vi "Phasor Explorer Refresh Settings.vi"(8 "error in (no error)":errorcluster, 11 "VI in":refnum<vi>) -> (0 "error out":errorcluster)   [LabVIEW 2019]
uses:
  Phasor Explorer Phasor Parameters.ctl
  Phasor Calculation Type.ctl
  SEPL Type.ctl
  Phasor Explorer Gate Parameters.ctl
  Gate Type.ctl
  Type of User-defined Function.ctl
  Phasor Explorer Decay Parameters.ctl
  IRF Model.ctl
  Phasor Explorer Display Parameters.ctl
  Type of Series.ctl
panel:
  in  "Display Parameters":T1={"# Points"=1, "Ramp Type"=enum."Linear", "Type of Series"=enum."1-Exp Decays", "Min tau"=0.0, "Max tau"=0.0, "Include 0"=FALSE, "Include Infinity"=FALSE} {"Min tau" min=0.0; "Max tau" min=0.0; "# Points" min=1 step=1}
  in  "Decay & IRF Parameters":T3 {"Lifetime" min=0.0; "IRF Period" min=0.0}
  in  "Gate Parameters":T5={"First Gate Start"=0.0, "Use Gate Center"=FALSE, "Gate Width"=0.0, "Gate Step"=0.0, "# Gates"=1.0, "Gate Type"=enum."Square", "Edge Width"=0.0, "Top Slope"=0.0, "Reversed Sawtooth?"=FALSE, "Analytical Computation"=FALSE, "Integration"=enum."Item 0", "Tolerance"=1.0, "# Steps"=1.0, "Type of User-defined Function"=enum."Gate", "Use Gate Step"=FALSE} {"# Steps" min=0.0; "Tolerance" min=0.0; "Top Slope" min=0.0; "Edge Width" min=0.0; "Gate Step" min=0.0; "# Gates" min=1.0 step=1.0; "Gate Width" min=0.0}
  in  "Phasor Parameters":T8={"Harmonic Frequency"=0.0, "Use f* = 1/D Frequency"=FALSE, "Calibrated Phasor"=FALSE, "Calibration Lifetime"=1e-09, "Phasor Calculation"=enum."Direct Sum", "SEPL Type"=enum."UC", "# Gates"=1.0, "Square Gate Width"=1e-09, "Show Ticks"=FALSE} {"Square Gate Width" min=0.0; "# Gates" min=0.0; "Calibration Lifetime" min=0.0; "Harmonic Frequency" min=0.0}
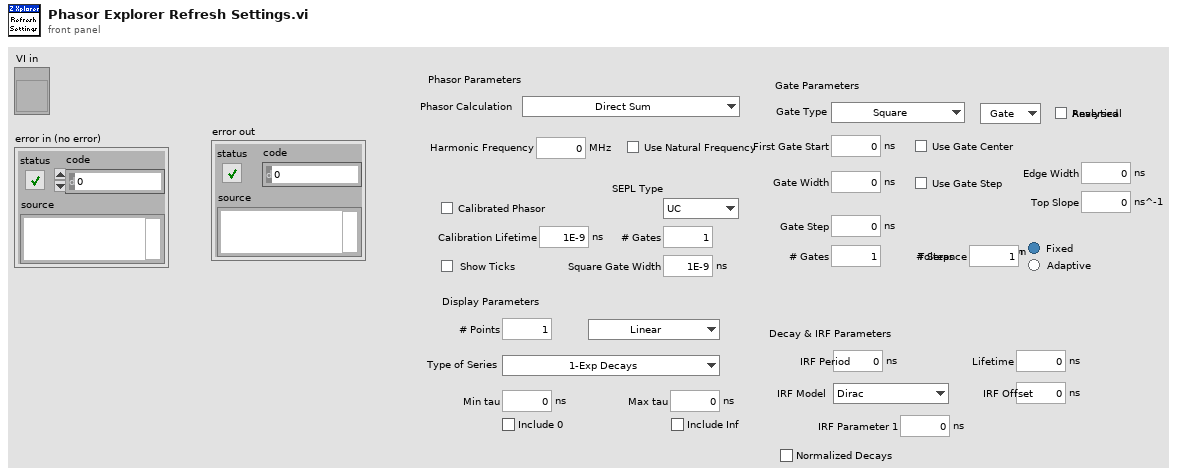
[diagram p1: front panel]
types:
  T1 = typedef "Phasor Explorer Display Parameters.ctl" = cluster{"# Points":i32, "Ramp Type":enum16{"Linear", "Logarithmic"}, "Type of Series":T2, "Min tau":dbl[unit], "Max tau":dbl[unit], "Include 0":bool, "Include Infinity":bool}
  T2 = typedef "Type of Series.ctl" = enum16{"1-Exp Decays", "Linear Combination of 1-Exp"}
  T3 = typedef "Phasor Explorer Decay Parameters.ctl" = cluster{"Lifetime":dbl[unit], "IRF Offset":dbl[unit], "IRF Period":dbl[unit], "Normalized Decays":bool, "IRF Model":T4, "IRF Parameter 1":dbl[unit]}
  T4 = typedef "IRF Model.ctl" = enum16{"Dirac", "Exponential"}
  T5 = typedef "Phasor Explorer Gate Parameters.ctl" = cluster{"First Gate Start":dbl[unit], "Use Gate Center":bool, "Gate Width":dbl[unit], "Gate Step":dbl[unit], "# Gates":dbl, "Gate Type":T6, "Edge Width":dbl[unit], "Top Slope":dbl[unit], "Reversed Sawtooth?":bool, "Analytical Computation":bool, "Integration":enum32{"Item 0", "Item 1"}, "Tolerance":dbl, "# Steps":dbl, "Type of User-defined Function":T7, "Use Gate Step":bool}
  T6 = typedef "Gate Type.ctl" = enum16{"Square", "Finite Edge Square", "Finite Edge, Tilted Top Square", "Triangle", "Sawtooth", "User-defined"}
  T7 = typedef "Type of User-defined Function.ctl" = enum16{"Gate", "IRF"}
  T8 = typedef "Phasor Explorer Phasor Parameters.ctl" = cluster{"Harmonic Frequency":dbl[unit], "Use f* = 1/D Frequency":bool, "Calibrated Phasor":bool, "Calibration Lifetime":dbl[unit], "Phasor Calculation":T9, "SEPL Type":T10, "# Gates":dbl, "Square Gate Width":dbl[unit], "Show Ticks":bool}
  T9 = typedef "Phasor Calculation Type.ctl" = enum16{"Direct Sum", "Analytical Formula"}
  T10 = typedef "SEPL Type.ctl" = enum16{"UC", "L_N", "L_N[W]", "L_X"}
  T11 = typedef "Phasor Explorer Settings List.ctl" = enum16{"Display Parameters", "Phasor Parameters", "Decay & IRF Parameters", "Gate Parameters", "Detector Parameters", "f*", "tau*"}
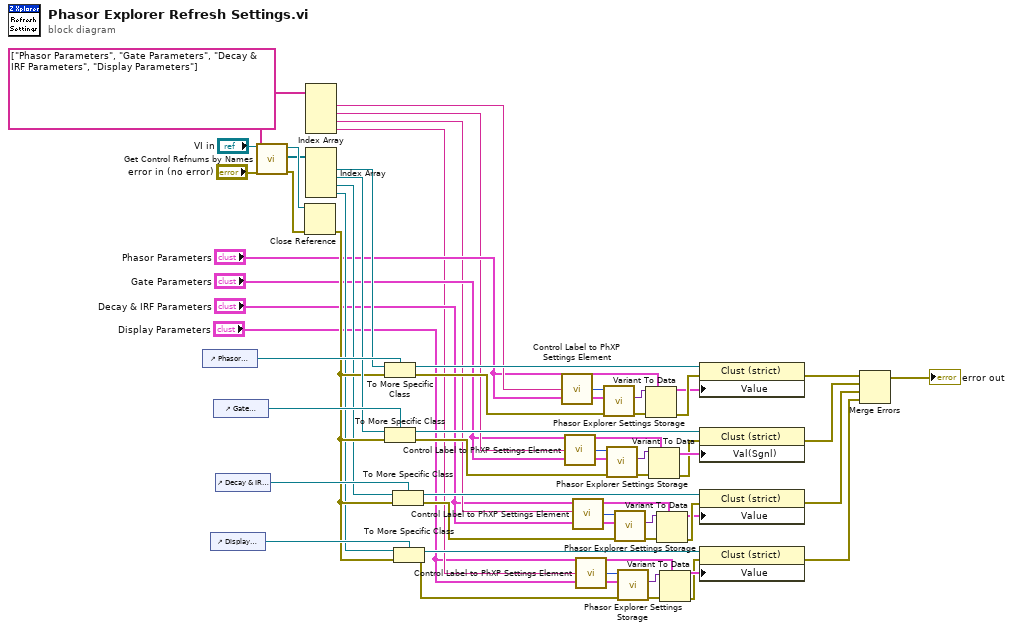
[diagram p0: block diagram]
diagram:
  w40 = string[] ["Phasor Parameters", "Gate Parameters", "Decay & IRF Parameters", "Display Parameters"] ("Control Labels")
  n1 = control-ref of="Phasor Parameters"() -> (w52:refnum<vi>)
  n2 = control-ref of="Display Parameters"() -> (w44:refnum<vi>)
  n3 = control-ref of="Gate Parameters"() -> (w51:refnum<vi>)
  n4 = control-ref of="Decay & IRF Parameters"() -> (w46:refnum<vi>)
  n5 = call "Get Control Refnums by Names.vi"("error in"="error in (no error)", "Control Labels"=w40, "VI  Ref"="VI in") -> ("error out"=w42:errorcluster, "Ctl Refnums"=w53:refnum<vi>[], "VI  Ref (out)"=w54:refnum<vi>)  [unwired: 5 in, 1 out]
  n6 = Close Reference(reference=w54, error in (no error)=w42) -> (error out=w41:errorcluster)
  n7 = Index Array(array=w40) -> (element #1=w34:string, element #2=w25:string, element #3=w16:string, element #4=w7:string)  [unwired: 4 in]
  n8 = Index Array(array=w53) -> (element #1=w48:refnum<vi>, element #2=w47:refnum<vi>, element #3=w39:refnum<vi>, element #4=w38:refnum<vi>)  [unwired: 4 in]
  n9 = To More Specific Class(target class=w52, reference=w48, error in=w41) -> (specific class reference=w50:refnum<vi>, error out=w26:errorcluster)
  n10 = To More Specific Class(target class=w51, reference=w47, error in=w41) -> (specific class reference=w49:refnum<vi>, error out=w24:errorcluster)
  n11 = To More Specific Class(target class=w46, reference=w39, error in=w41) -> (specific class reference=w45:refnum<vi>, error out=w14:errorcluster)
  n12 = To More Specific Class(target class=w44, reference=w38, error in=w41) -> (specific class reference=w43:refnum<vi>, error out=w9:errorcluster)
  n13 = call "Control Label to PhXP Settings Element.vi"("Label.Text"=w34) -> ("Settings List Element"=w35:T11)
  n14 = call "Control Label to PhXP Settings Element.vi"("Label.Text"=w25) -> ("Settings List Element"=w30:T11)
  n15 = call "Control Label to PhXP Settings Element.vi"("Label.Text"=w16) -> ("Settings List Element"=w19:T11)
  n16 = call "Control Label to PhXP Settings Element.vi"("Label.Text"=w7) -> ("Settings List Element"=w13:T11)
  n17 = call "Phasor Explorer Settings Storage.vi"("Error In"=w26, "Variant Data in"="Phasor Parameters", "Settings List"=w35) -> ("Error Out"=w36:errorcluster, "Variant Data out"=w37:variant)  [unwired: 7 in]
  n18 = call "Phasor Explorer Settings Storage.vi"("Error In"=w24, "Variant Data in"="Gate Parameters", "Settings List"=w30) -> ("Error Out"=w29:errorcluster, "Variant Data out"=w28:variant)  [unwired: 7 in]
  n19 = call "Phasor Explorer Settings Storage.vi"("Error In"=w14, "Variant Data in"="Decay & IRF Parameters", "Settings List"=w19) -> ("Error Out"=w20:errorcluster, "Variant Data out"=w21:variant)  [unwired: 7 in]
  n20 = call "Phasor Explorer Settings Storage.vi"("Error In"=w9, "Variant Data in"="Display Parameters", "Settings List"=w13) -> ("Error Out"=w12:errorcluster, "Variant Data out"=w11:variant)  [unwired: 7 in]
  n21 = Variant To Data(error in=w36, type="Phasor Parameters", Variant=w37) -> (data=w32:T8, error out=w33:errorcluster)
  n22 = Variant To Data(error in=w29, type="Gate Parameters", Variant=w28) -> (data=w27:T5, error out=w23:errorcluster)
  n23 = Variant To Data(error in=w20, type="Decay & IRF Parameters", Variant=w21) -> (data=w17:T3, error out=w18:errorcluster)
  n24 = Variant To Data(error in=w12, type="Display Parameters", Variant=w11) -> (data=w10:T1, error out=w8:errorcluster)
  n25 = property class="Clust (strict)"(reference=w50, error in=w33, "Value"=w32) -> (error out=w5:errorcluster)  [unwired: 1 out]
  n26 = property class="Clust (strict)"(reference=w49, error in=w23, "Val(Sgnl)"=w27) -> (error out=w4:errorcluster)  [unwired: 1 out]
  n27 = property class="Clust (strict)"(reference=w45, error in=w18, "Value"=w17) -> (error out=w3:errorcluster)  [unwired: 1 out]
  n28 = property class="Clust (strict)"(reference=w43, error in=w8, "Value"=w10) -> (error out=w2:errorcluster)  [unwired: 1 out]
  n29 = Merge Errors(w5, w4, w3, w2) -> (→"error out":errorcluster)
